vi "C4209 Create-Delete.vi"(0 "Reference in":refnum<k7>, 1 "Channel (1)":i32=1, 2 "Mode (0: Create)":u16(ring) items=["Create", "Delete", "Select", "Delete All"], 3 "error in":errorcluster, 4 "Measurements":i32[](array[ring])=[0, 1, 2, 3] items=["S11", "S21", "S12", "S22", "A", "B", "R1", "R2", "A/B", "B/A"], 5 "Measurement Name":string) -> (7 "Reference out":refnum<k7>, 10 "Error Out":errorcluster)   [LabVIEW 2019, in "C4209 PNA.lvclass"]
uses:
  C4209 PNA.lvclass
  <instrlib>/CMT S2 Series VNA/CMT S2 Series VNA.lvlib
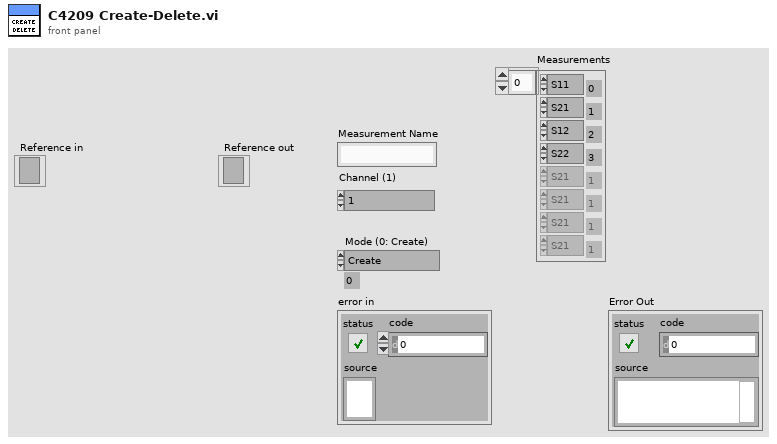
[diagram p1: front panel]
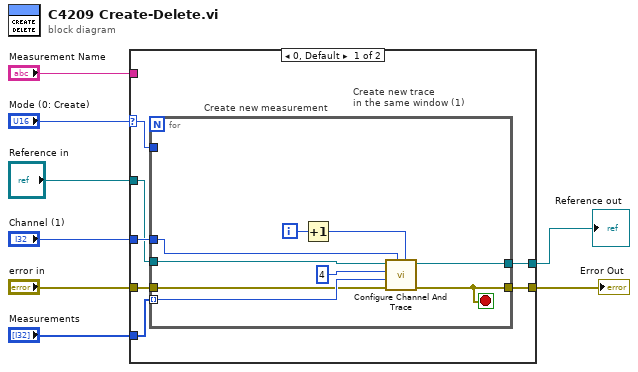
[diagram p0: block diagram]
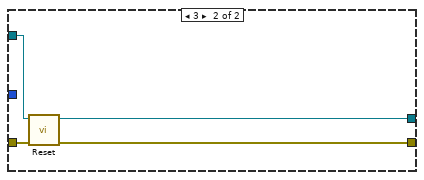
[diagram p2: hidden frame]
diagram:
  n1 = case shown="0, Default" "Mode (0: Create)" {
    selector: "Mode (0: Create)" -> [w11 _]
    tunnel: "Reference in" -> [w10 w27]
    tunnel: "Measurements" -> [w15 _]
    tunnel: "Measurement Name" -> [_ _]
    tunnel: "Channel (1)" -> [w14 _]
    tunnel: [w13 w25] -> w5
    tunnel: "error in" -> [w12 w26]
    tunnel: [w9 w28] -> w1
    frame 0, Default {
      # "Create new trace\nin the same window (1)"
      # "Create new measurement"
      n2 = for {
        tunnel: w15 -> [w20] mode=indexing
        tunnel: w14 -> [w23]
        tunnel: [w18] -> w13
        tunnel: w12 -> [w19]
        tunnel: w11 -> [_]
        tunnel: w10 -> [w21]
        tunnel: [w17] -> w9
        i -> [w24]
        stop <- w18 stop-if-true
        n3 = Increment(x=w24) -> (x+1=w22:i32)
        n4 = call <instrlib>:"Configure Channel And Trace.vi"("Active Trace (1)"=w22, "Active Channel (1)"=w23, "error in (no error)"=w19, "Measurement Parameter (0: S11)"=w20, "Number of Traces (1)"=4, "Reference in"=w21) -> ("error out"=w18:errorcluster, "Reference out"=w17:refnum<k7>)  [unwired: 4 in]
      }
    }
    frame 3 {
      n5 = call <instrlib>:"Reset.vi"("error in (no error)"=w26, "Reference in"=w27) -> ("error out"=w25:errorcluster, "Reference out"=w28:refnum<k7>)  [unwired: 8 in]
    }
  }
  "Error Out" <- w5
  "Reference out" <- w1
